vi "Write AIP Status.vi"(7 "AIP Depth Min":u8, 8 "error in (no error)":errorcluster, 9 "Raw Frame":refnum<class "RDS Serial Frame.lvclass">, 10 "AIP Status":T1, 11 "AIP Status Response in":refnum<class "AIP Status Response.lvclass">) -> (0 "error out":errorcluster, 3 "AIP Status Response out":refnum<class "AIP Status Response.lvclass">)   [LabVIEW 2015, in "RDS Child Messages.lvlib" / "AIP Status Response.lvclass"]
uses:
  AIP Status Response.lvclass
  RDS Instruments/AIP/AIP Status.ctl
  RDS Instruments/AIP/AIP States.ctl
  RDS Serial Handler/RDS Serial Frame.lvclass
  AIP Status Response.lvclass/AIP Status Response.ctl
  RDS Instruments/RDS Instrument Library.lvlib
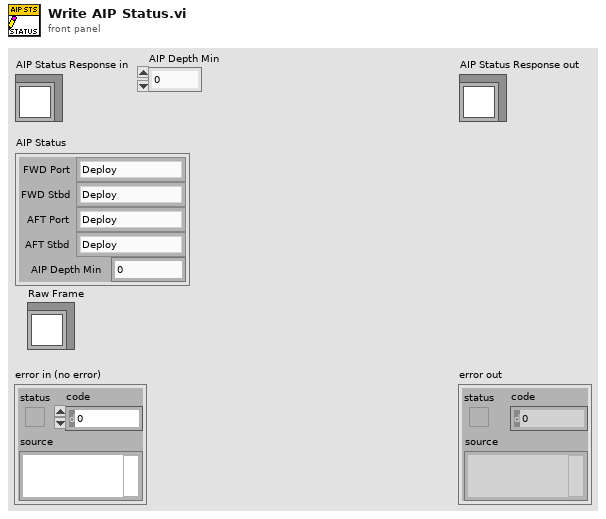
[diagram p1: front panel]
types:
  T1 = typedef "RDS Instrument Library.lvlib/AIP Status.ctl" = cluster{"FWD Port":T2, "FWD Stbd":T2, "AFT Port":T2, "AFT Stbd":T2, "AIP Depth Min":u8}
  T2 = typedef "RDS Instrument Library.lvlib/AIP States.ctl" = enum16{"Deploy", "Deploying", "Deployed", "Stow", "Stowing", "Stowed", "Fault", "brakeOnStow", "breakOnDeploy", "Stopped", "Stopping"}
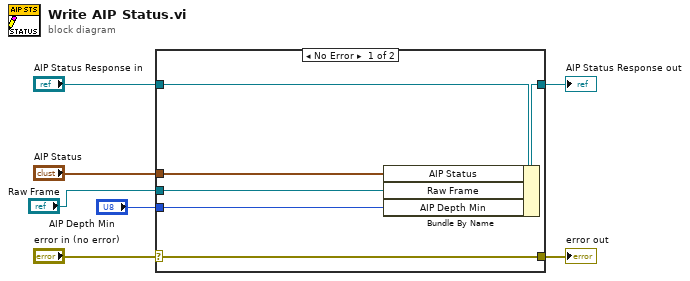
[diagram p0: block diagram]
diagram:
  n1 = case shown="No Error" "error in (no error)" {
    selector: "error in (no error)" -> [w13 w14]
    tunnel: [w13 w14] -> w6
    tunnel: [w11 w15] -> w4
    tunnel: "AIP Status Response in" -> [w12 w15]
    tunnel: "AIP Status" -> [w10 _]
    tunnel: "Raw Frame" -> [w9 _]
    tunnel: "AIP Depth Min" -> [w8 _]
    frame No Error {
      n2 = Bundle By Name(cluster=w12, "AIP Status"=w10, "Raw Frame"=w9, "AIP Depth Min"=w8) -> (w11:refnum<class "AIP Status Response.lvclass">)
    }
    frame Error {
    }
  }
  "error out" <- w6
  "AIP Status Response out" <- w4
